vi "Refresh Controls.vi"(8 "error in":errorcluster, 11 "Base Software in":refnum<class "Main.lvclass">) -> (0 "error out":errorcluster, 3 "Base Software out":refnum<class "Main.lvclass">)   [LabVIEW 2023, in "Main.lvlib" / "Main.lvclass"]
uses:
  Project/Main.lvclass
  Project/Main.lvclass/Main.ctl
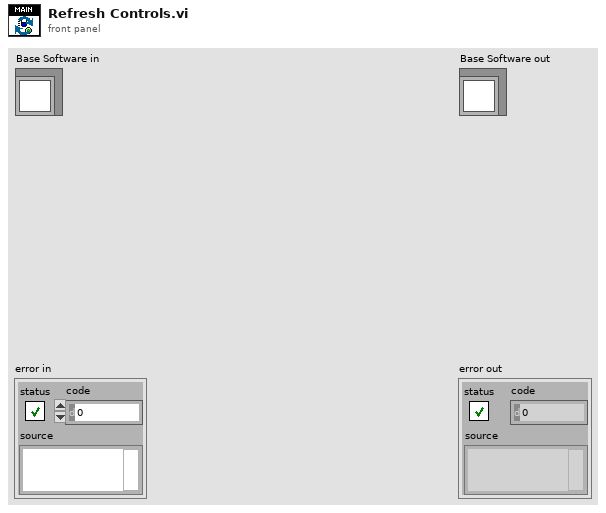
[diagram p1: front panel]
types:
  T1 = enum8{"Enabled", "Disabled", "Disabled and Grayed Out"}
  T2 = typedef "Engine.lvlibp/Engine.lvclass/System Status.ctl" = enum16{"Logged Off", "UUT_Info_Missing", "Idle", "Error", "Warning", "Loading", "Config", "Manual", "Automation", "Report_View", "Previous"}
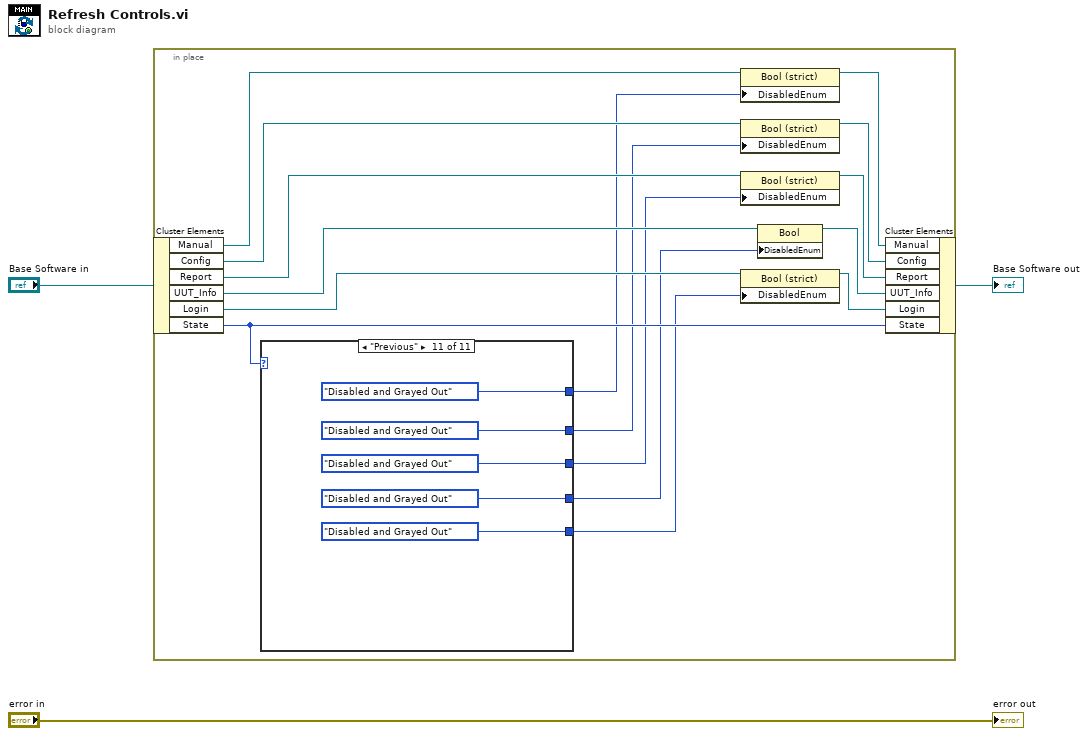
[diagram p0: block diagram]
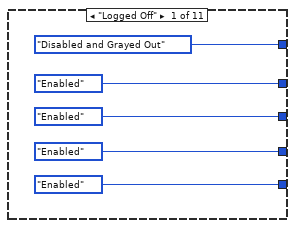
[diagram p2: hidden frame]
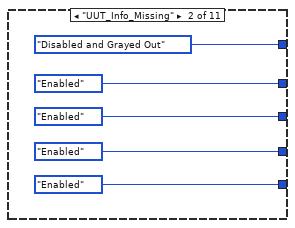
[diagram p3: hidden frame]
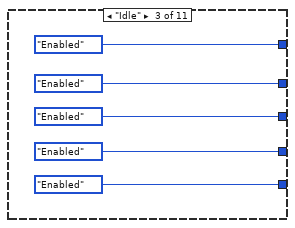
[diagram p4: hidden frame]
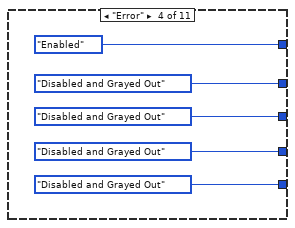
[diagram p5: hidden frame]
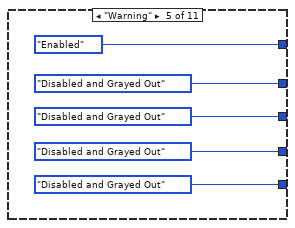
[diagram p6: hidden frame]
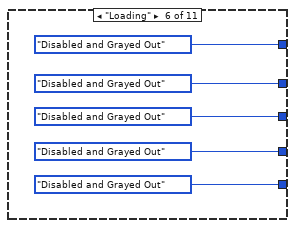
[diagram p7: hidden frame]
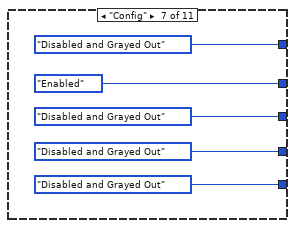
[diagram p8: hidden frame]
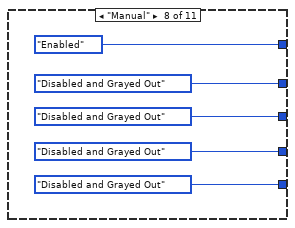
[diagram p9: hidden frame]
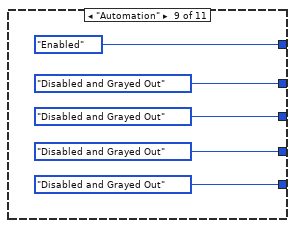
[diagram p10: hidden frame]
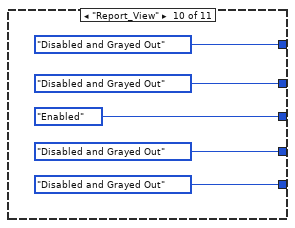
[diagram p11: hidden frame]
diagram:
  n1 = in-place {
    n2 = in-place-cluster #1("Base Software in") -> ("Manual"=w13:refnum<vi>, "Config"=w14:refnum<vi>, "Report"=w15:refnum<vi>, "UUT_Info"=w16:refnum<vi>, "Login"=w18:refnum<vi>, "State"=w19:T2)
    n3 = case shown="\"Previous\"" w19 {
      tunnel: [T1."Disabled and Grayed Out" ("Disabled") T1."Disabled and Grayed Out" ("Disabled") T1."Enabled" ("Disabled") T1."Enabled" ("Disabled") T1."Enabled" ("Disabled") T1."Disabled and Grayed Out" ("Disabled") T1."Disabled and Grayed Out" ("Disabled") T1."Enabled" ("Disabled") T1."Enabled" ("Disabled") T1."Disabled and Grayed Out" ("Disabled") T1."Disabled and Grayed Out" ("Disabled")] -> w8
      tunnel: [T1."Enabled" ("Disabled") T1."Enabled" ("Disabled") T1."Enabled" ("Disabled") T1."Disabled and Grayed Out" ("Disabled") T1."Disabled and Grayed Out" ("Disabled") T1."Disabled and Grayed Out" ("Disabled") T1."Enabled" ("Disabled") T1."Disabled and Grayed Out" ("Disabled") T1."Disabled and Grayed Out" ("Disabled") T1."Disabled and Grayed Out" ("Disabled") T1."Disabled and Grayed Out" ("Disabled")] -> w7
      tunnel: [T1."Enabled" ("Disabled") T1."Enabled" ("Disabled") T1."Enabled" ("Disabled") T1."Disabled and Grayed Out" ("Disabled") T1."Disabled and Grayed Out" ("Disabled") T1."Disabled and Grayed Out" ("Disabled") T1."Disabled and Grayed Out" ("Disabled") T1."Disabled and Grayed Out" ("Disabled") T1."Disabled and Grayed Out" ("Disabled") T1."Enabled" ("Disabled") T1."Disabled and Grayed Out" ("Disabled")] -> w6
      tunnel: [T1."Enabled" ("Disabled") T1."Enabled" ("Disabled") T1."Enabled" ("Disabled") T1."Disabled and Grayed Out" ("Disabled") T1."Disabled and Grayed Out" ("Disabled") T1."Disabled and Grayed Out" ("Disabled") T1."Disabled and Grayed Out" ("Disabled") T1."Disabled and Grayed Out" ("Disabled") T1."Disabled and Grayed Out" ("Disabled") T1."Disabled and Grayed Out" ("Disabled") T1."Disabled and Grayed Out" ("Disabled")] -> w5
      tunnel: [T1."Enabled" ("Disabled") T1."Enabled" ("Disabled") T1."Enabled" ("Disabled") T1."Disabled and Grayed Out" ("Disabled") T1."Disabled and Grayed Out" ("Disabled") T1."Disabled and Grayed Out" ("Disabled") T1."Disabled and Grayed Out" ("Disabled") T1."Disabled and Grayed Out" ("Disabled") T1."Disabled and Grayed Out" ("Disabled") T1."Disabled and Grayed Out" ("Disabled") T1."Disabled and Grayed Out" ("Disabled")] -> w4
      frame "Logged Off" {
      }
      frame "UUT_Info_Missing" {
      }
      frame "Idle" {
      }
      frame "Error" {
      }
      frame "Warning" {
      }
      frame "Loading" {
      }
      frame "Config" {
      }
      frame "Manual" {
      }
      frame "Automation" {
      }
      frame "Report_View" {
      }
      frame "Previous" {
      }
    }
    n4 = property class="Bool (strict)"(reference=w13, "DisabledEnum"=w8) -> (reference out=w9:refnum<vi>)  [unwired: 1 in, 1 out]
    n5 = property class="Bool (strict)"(reference=w14, "DisabledEnum"=w7) -> (reference out=w10:refnum<vi>)  [unwired: 1 in, 1 out]
    n6 = property class="Bool (strict)"(reference=w15, "DisabledEnum"=w6) -> (reference out=w11:refnum<vi>)  [unwired: 1 in, 1 out]
    n7 = property class="Bool (strict)"(reference=w18, "DisabledEnum"=w4) -> (reference out=w17:refnum<vi>)  [unwired: 1 in, 1 out]
    n8 = property class="Bool"(reference=w16, "DisabledEnum"=w5) -> (reference out=w12:refnum<vi>)  [unwired: 1 in, 1 out]
    n9 = in-place-cluster #1("Manual"=w9, "Config"=w10, "Report"=w11, "UUT_Info"=w12, "Login"=w17, "State"=w19) -> (→"Base Software out":refnum<class "Main.lvclass">)
  }
  "error out" <- "error in"
